vi "Serial Output Test.vi"() -> ()   [LabVIEW 2011]
doc: "Just tests whether we get any data out of the serial port and shows what data we get. Requires the user to select the port the serial is hooked up to."
uses:
  <vilib>/Instr/_visa.llb/VISA Configure Serial Port (Instr).vi
panel:
  in  "Serial Port":refnum<visa-resource-name>
  out "# of bytes read":u32
  in  "stop":bool
  out "Data read (numeric)":u8[](array[numeric])
  out "Data read (string)":string
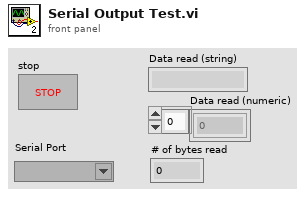
[diagram p1: front panel]
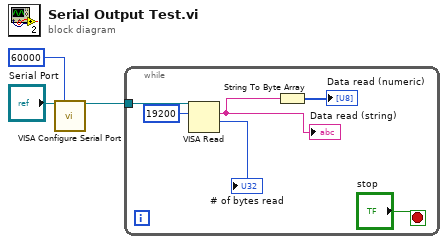
[diagram p0: block diagram]
diagram:
  n1 = call-poly "VISA Configure Serial Port"("VISA resource name"="Serial Port", "timeout (10sec)"=u32 60000) -> ("VISA resource name out"=w1:refnum<visa-resource-name>)  [unwired: 12 in, 1 out]
  n2 = while {
    tunnel: w1 -> [w4]
    stop <- "stop" stop-if-true
    n3 = VISA Read(VISA resource name=w4, byte count=u32 19200) -> (read buffer=w8:string, return count=→"# of bytes read":u32)  [unwired: 1 in, 2 out]
    "Data read (string)" <- w8
    n4 = String To Byte Array(string=w8) -> (unsigned byte array=→"Data read (numeric)":u8[])
  }
